vi "Close Remote uService GUI.vi"(8 "error in (no error)":errorcluster, 11 "Remote GUI":refnum<vi>) -> (0 "error out":errorcluster, 3 "reference out":refnum<vi>)   [LabVIEW 2026, in "TALOS.lvlib" / "Common GUI v3.lvlib"]
uses:
  Common GUI v3.lvlib
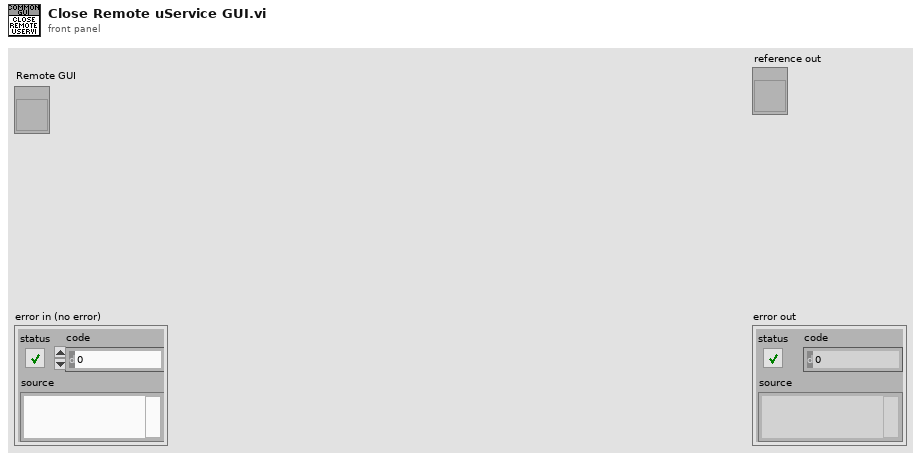
[diagram p1: front panel]
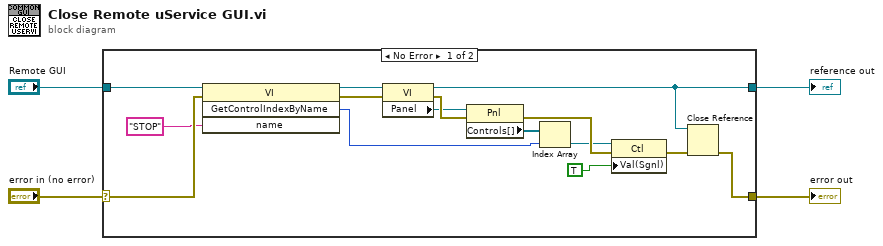
[diagram p0: block diagram]
diagram:
  n1 = case shown="No Error" "error in (no error)" {
    selector: "error in (no error)" -> [w6 w21]
    tunnel: "Remote GUI" -> [w18 w20]
    tunnel: [w9 w20] -> w3
    tunnel: [w7 w21] -> w2
    frame No Error {
      n2 = invoke class="VI" method="GetControlIndexByName"(reference=w18, error in=w6, "name"="STOP" ("Control Name")) -> (reference out=w17:refnum<vi>, error out=w16:errorcluster, "GetControlIndexByName"=w12:i32)  [unwired: 1 in, 1 out]
      n3 = property class="VI"(reference=w17, error in=w16) -> (reference out=w9:refnum<vi>, error out=w15:errorcluster, "Panel"=w14:refnum<vi>)
      n4 = property class="Pnl"(reference=w14, error in=w15) -> (error out=w19:errorcluster, "Controls[]"=w13:refnum<vi>[])  [unwired: 1 out]
      n5 = Index Array(array=w13, index=w12) -> (element=w11:refnum<vi>)
      n6 = property class="Ctl"(reference=w11, error in=w19, "Val(Sgnl)"=TRUE) -> (error out=w8:errorcluster)  [unwired: 1 out]
      n7 = Close Reference(reference=w9, error in (no error)=w8) -> (error out=w7:errorcluster)
    }
    frame Error {
    }
  }
  "error out" <- w2
  "reference out" <- w3
